vi "Write Network Protocol.vi"(8 "error in (no error)":errorcluster, 10 "Network Protocol":refnum<class "Network Protocol.lvclass">, 11 "Master CR in":refnum<class "Master CR.lvclass">) -> (0 "error out":errorcluster, 3 "Master CR out":refnum<class "Master CR.lvclass">)   [LabVIEW 2021, in "Master CR.lvclass"]
uses:
  Master CR.lvclass
  Modbus_v121c/Network Protocol/Network Protocol.lvclass
  Master CR.lvclass/Master CR.ctl
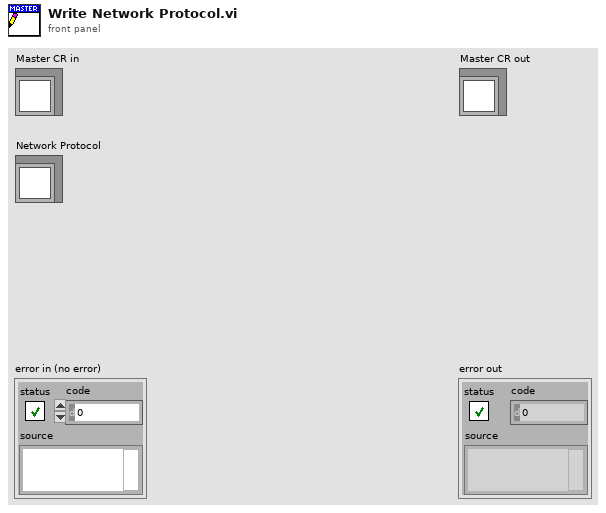
[diagram p1: front panel]
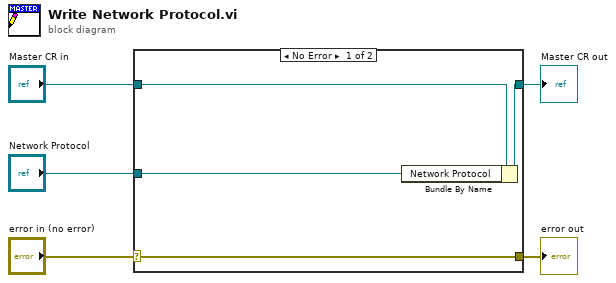
[diagram p0: block diagram]
diagram:
  n1 = case shown="No Error" "error in (no error)" {
    selector: "error in (no error)" -> [w9 w10]
    tunnel: [w9 w10] -> w4
    tunnel: [w7 w11] -> w2
    tunnel: "Master CR in" -> [w8 w11]
    tunnel: "Network Protocol" -> [w6 _]
    frame No Error {
      n2 = Bundle By Name(cluster=w8, "Network Protocol"=w6) -> (w7:refnum<class "Master CR.lvclass">)
    }
    frame Error {
    }
  }
  "error out" <- w4
  "Master CR out" <- w2
